vi "AH 2550 Continuous Measurement.vi"() -> ()   [LabVIEW 2016]
doc: "This example shows how to configure the bridge,initiate continuous capacitance measurement, read the results from the bridge, and parse the measurement results."
uses:
  Andeen-Hagerling 2550.lvlib
panel:
  in  "Interval":dbl min=0.0 max=99999999.0 step=0.1 format="%#_10f"
  out "Loss Chart":dbl(graph)
  out "Capacitance Chart":dbl(graph)
  out "Sample Switch":i32
  in  "stop":bool
  out "Frequency":dbl
  out "Units Display":i32(ring)=1 items=["nanosiemens"=1, "dissipation factor"=2, "kilohms"=3, "gigohms"=4, "loss vector (jpF)"=5]
  out "Error Code":i32
  out "Applied Voltage":dbl format="%#_6f"
  out "Loss":dbl
  out "Capacitance":dbl format="%#_10f"
  in  "Units":i32(ring)=1 items=["nanosiemens"=1, "dissipation factor"=2, "kilohms"=3, "gigohms"=4, "loss vector (jpF)"=5]
  in  "Maximum Voltage":dbl=15.0 min=0.0003 max=15.0 step=1.0 format="%#.6f"
  in  "Average Exponent":u16=4 max=15
  in  "VISA resource name":refnum<visa-resource-name>
  in  "Serial Configuration":T1={"Baud Rate"=9600, "Parity"=0, "Data Bits"=8, "Stop Bits"=10} {"Stop Bits" items=["1.0"=10, "1.5"=15, "2.0"=20]; "Data Bits" items=["7"=7, "8"=8]; "Parity" items=["None", "Odd", "Even", "Mark", "Space"]; "Baud Rate" items=["300"=300, "600"=600, "1200"=1200, "2400"=2400, "4800"=4800, "9600"=9600, "19200"=19200]}
  # "AH 2550A ULTRA-PRECISION 1kHz CAPACITANCE BRIDGE"
  # "Continuous Measurement"
  # "Measurement Parameters"
  # "Measurement Results"
  # "picoFarads"
  # "V"
  # "Continuous Parameters"
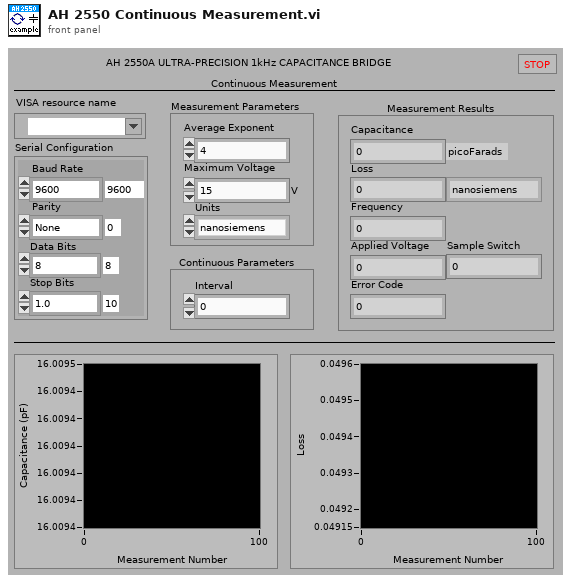
[diagram p1: front panel]
types:
  T1 = cluster{"Baud Rate":u32, "Parity":u16, "Data Bits":u16, "Stop Bits":u16}
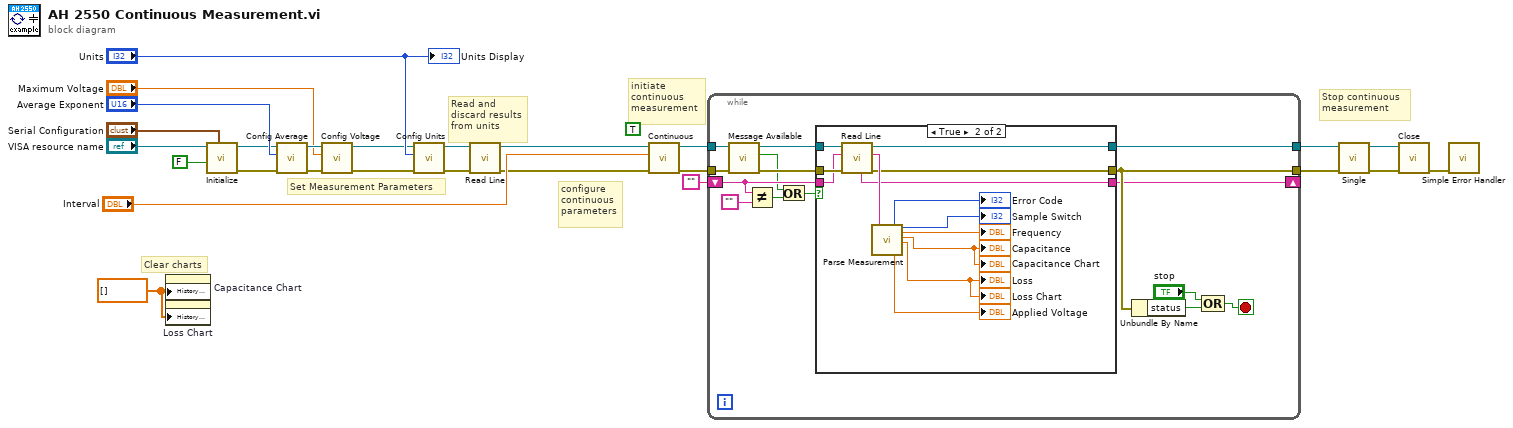
[diagram p0: block diagram]
diagram:
  w12 = dbl[] [] ("History Data")
  (unwired) TRUE ("On (true)")
  # "configure\ncontinuous\nparameters"
  # "Clear charts"
  # "Stop continuous\nmeasurement"
  # "initiate\ncontinuous\nmeasurement"
  # "Set Measurement Parameters"
  # "Read and\ndiscard results\nfrom units"
  n1 = property on="Capacitance Chart" class="WFChart (strict)"("History Data"=w12) -> ()  [unwired: 2 in, 2 out]
  n2 = property on="Loss Chart" class="WFChart (strict)"("History Data"=w12) -> ()  [unwired: 2 in, 2 out]
  n3 = call "Initialize.vi"("Serial Configuration"="Serial Configuration", "Reset (True)"=FALSE, "VISA resource name"="VISA resource name") -> ("error out"=w17:errorcluster, "VISA resource name out"=w18:refnum<visa-resource-name>)  [unwired: 7 in]
  n4 = call "Config Average.vi"("error in"=w17, "Average Exponent (4)"="Average Exponent", "VISA resource name"=w18) -> ("error out"=w23:errorcluster, "VISA resource name out"=w24:refnum<visa-resource-name>)  [unwired: 7 in]
  n5 = call "Config Voltage.vi"("error in"=w23, "Voltage (15 V)"="Maximum Voltage", "VISA resource name"=w24) -> ("error out"=w6:errorcluster, "VISA resource name out"=w7:refnum<visa-resource-name>)  [unwired: 7 in]
  n6 = call "Config Units.vi"("error in"=w6, "Units (nS)"="Units", "VISA resource name"=w7) -> ("error out"=w19:errorcluster, "VISA resource name out"=w20:refnum<visa-resource-name>)  [unwired: 7 in]
  n7 = call "Read Line.vi"("error in"=w19, "VISA resource name"=w20) -> ("error out"=w9:errorcluster, "VISA resource name out"=w8:refnum<visa-resource-name>)  [unwired: 5 in, 3 out]
  n8 = call "Continuous.vi"("error in"=w9, "Interval (0)"="Interval", "VISA resource name"=w8) -> ("error out"=w14:errorcluster, "VISA resource name out"=w15:refnum<visa-resource-name>)  [unwired: 7 in]
  n9 = while {
    tunnel: [w41] -> w5
    tunnel: [w40] -> w2
    tunnel: w15 -> [w38]
    tunnel: w14 -> [w36]
    shift-right: [w39] -> _
    shift-left: "" -> [w30]
    stop <- w33 stop-if-true
    n10 = call "Message Available.vi"("error in"=w36, "VISA resource name"=w38) -> ("error out"=w35:errorcluster, "message available"=w28:bool, "VISA resource name out"=w37:refnum<visa-resource-name>)  [unwired: 7 in]
    n11 = Not Equal?(x=w30, y="") -> (x != y?=w29:bool)
    n12 = Or(x=w28, y=w29) -> (x .or. y?=w27:bool)
    n13 = case shown="True" w27 {
      tunnel: [w44 w57] -> w41
      tunnel: w37 -> [w44 w55]
      tunnel: w35 -> [w43 w54]
      tunnel: [w43 w50] -> w40
      tunnel: [w42 w47] -> w39
      tunnel: w30 -> [w42 w46]
      frame False {
      }
      frame True {
        n14 = call "Read Line.vi"("error in"=w54, "Previous"=w46, "VISA resource name"=w55) -> ("error out"=w50:errorcluster, "Message"=w56:string, "VISA resource name out"=w57:refnum<visa-resource-name>, "Remaining"=w47:string)  [unwired: 4 in, 1 out]
        n15 = call "Parse Measurement.vi"("Measurement Line"=w56) -> ("Error Code"=→"Error Code":i32, "Voltage"=→"Applied Voltage":dbl, "Sample"=→"Sample Switch":i32, "Frequency"=→"Frequency":dbl, "Capacitance"=→"Capacitance" →"Capacitance Chart":dbl, "Loss"=→"Loss" →"Loss Chart":dbl)  [unwired: 10 in, 3 out]
      }
    }
    n16 = Unbundle By Name(w40) -> ("status"=w34:bool)
    n17 = Compound Arithmetic op=OR("stop", w34) -> (w33:bool)
  }
  n18 = call "Single.vi"("error in"=w2, "VISA resource name"=w5) -> ("error out"=w3:errorcluster, "VISA resource name out"=w4:refnum<visa-resource-name>)  [unwired: 8 in]
  n19 = call "Close.vi"("error in (no error)"=w3, "VISA resource name"=w4) -> ("error out"=w13:errorcluster)  [unwired: 9 in]
  n20 = call <vilib>:"Simple Error Handler.vi"("error in (no error)"=w13) -> ()  [unwired: 4 in, 5 out]
  "Units Display" <- "Units"
